vi "SerialLoopback.vi"(10 "Message to be Sent":string caption="String", 11 "VISA resource name":refnum<visa-resource-name>="loop://") -> ()   [LabVIEW 2014]
doc: "This examples shows the ideal design for a serial write/read VI running on the Raspberry Pi target. It uses the Raspberry Pi loopback serial address: loop://.\n\nThe VI is ready to run and doesn't require any external hardware connection. Type a value on the Message to be Sent Control and hit the SEND button. The same value will be displayed in the Message received indicator.\n\nSend stop message to stop the VI execution."
uses:
  <vilib>/Instr/_visa.llb/VISA Configure Serial Port (Instr).vi
panel:
  in  "Serial Settings":T1={"baud rate"=9600, "data bits"=8, "parity"=enum."None", "stop bits"=10, "flow control"=0} {"flow control" items=["None"=0, "XON/XOFF"=1, "RTS/CTS"=2, "DTR/DSR"=4]; "stop bits" items=["1.0"=10, "1.5"=15, "2.0"=20]; "data bits" min=5 max=8 step=1; "baud rate" items=["75"=75, "110"=110, "134"=134, "150"=150, "300"=300, "600"=600, "1200"=1200, "1800"=1800, "2400"=2400, "4800"=4800, "7200"=7200, "9600"=9600, "14400"=14400, "19200"=19200, "28800"=28800, "38400"=38400, "56000"=56000, "57600"=57600, "115200"=115200, "128000"=128000, "230400"=230400]}
  out "count":i32
  out "Message received":string
  in  "Send":bool
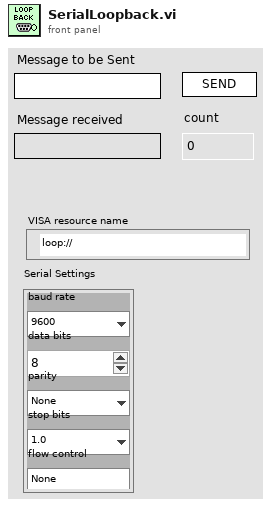
[diagram p1: front panel]
types:
  T1 = cluster{"baud rate":u32, "data bits":u16, "parity":enum16{"None", "Odd", "Even", "Mark", "Space"}, "stop bits":u16, "flow control":u16}
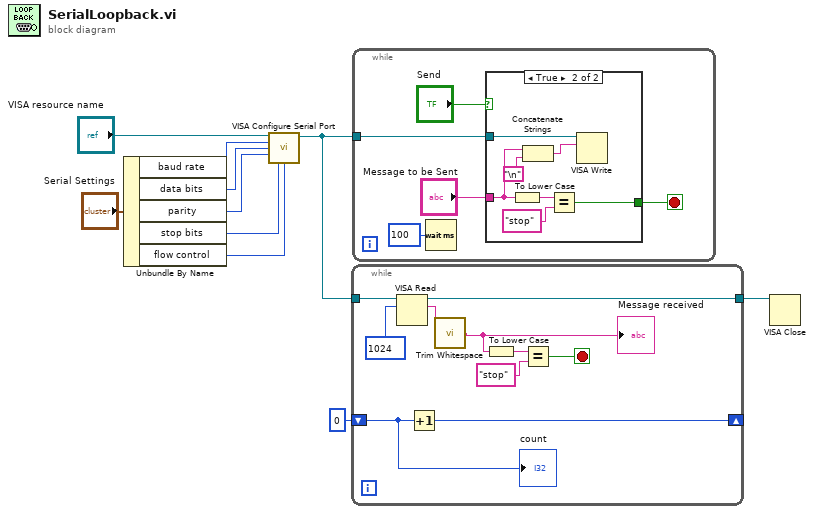
[diagram p0: block diagram]
diagram:
  n1 = Unbundle By Name("Serial Settings") -> ("baud rate"=w5:u32, "data bits"=w4:u16, "parity"=w3:enum16{"None", "Odd", "Even", "Mark", "Space"}, "stop bits"=w2:u16, "flow control"=w1:u16)
  n2 = call-poly "VISA Configure Serial Port"("VISA resource name"="VISA resource name", "baud rate (9600)"=w5, "data bits (8)"=w4, "parity (0:none)"=w3, "stop bits (10: 1 bit)"=w2, "flow control (0:none)"=w1) -> ("VISA resource name out"=w9:refnum<visa-resource-name>)  [unwired: 8 in, 1 out]
  n3 = while {
    shift-right: [w20] -> _
    shift-left: 0 -> [w16]
    tunnel: w9 -> [w15]
    tunnel: [w14] -> w8
    stop <- w17 stop-if-true
    n4 = VISA Read(VISA resource name=w15, byte count=u32 1024) -> (VISA resource name out=w14:refnum<visa-resource-name>, read buffer=w12:string)  [unwired: 1 in, 2 out]
    n5 = Increment(x=w16) -> (x+1=w20:i32)
    n6 = call <vilib>:"Trim Whitespace.vi"("string"=w12) -> ("trimmed string"=w11:string)  [unwired: 1 in]
    "Message received" <- w11
    n7 = To Lower Case(string=w11) -> (all lower case string=w19:string)
    n8 = Equal?(x=w19, y="stop") -> (x = y?=w17:bool)
    "count" <- w16
  }
  n9 = while {
    tunnel: w9 -> [w23]
    stop <- w21 stop-if-true
    n10 = Wait (ms)(milliseconds to wait=u32 100) -> ()  [unwired: 1 out]
    n11 = case shown="True" "Send" {
      tunnel: w23 -> [_ w30]
      tunnel: "Message to be Sent" -> [_ w28]
      tunnel: [_ w31] -> w21
      frame False {
      }
      frame True {
        n12 = To Lower Case(string=w28) -> (all lower case string=w29:string)
        n13 = Concatenate Strings(w28, "\n") -> (w27:string)
        n14 = Equal?(x=w29, y="stop") -> (x = y?=w31:bool)
        n15 = VISA Write(VISA resource name=w30, write buffer=w27) -> ()  [unwired: 1 in, 3 out]
      }
    }
  }
  n16 = VISA Close(VISA resource name=w8) -> ()  [unwired: 1 in, 1 out]
